vi "Range_Adjust.vi"(8 "error in (no error)":errorcluster, 11 ".NET Reference in":refnum<k24>) -> (0 "error out":errorcluster, 3 "Reference out":refnum<k24>)   [LabVIEW 2017]
doc: "OSU range adjust"
uses:
  D:/test/FULLband-sts/Fullband_Sample/DLL/InstrumentDLL.dll
  DLL/InstrumentDLL.dll
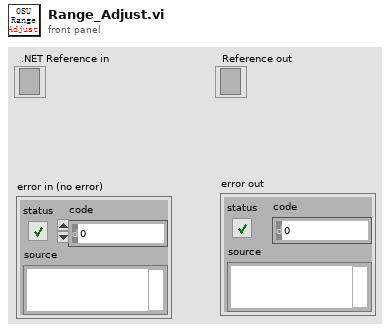
[diagram p1: front panel]
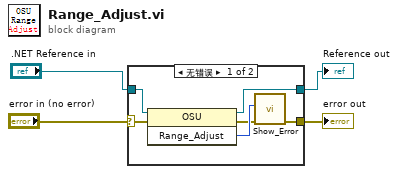
[diagram p0: block diagram]
diagram:
  n1 = case shown="无错误" "error in (no error)" {
    selector: "error in (no error)" -> [w8 w12]
    tunnel: ".NET Reference in" -> [w10 w11]
    tunnel: [w9 w11] -> w3
    tunnel: [w5 w12] -> w1
    frame No Error {
      n2 = invoke on="调用节点" class="OSU" method="Range_Adjust"(reference=w10, error in=w8) -> (reference out=w9:refnum<k24>, error out=w6:errorcluster, "Range_Adjust"=w7:i32)  [unwired: 1 in]
      n3 = call "Show_Error.vi"("error in (no error)"=w6, "Error"=w7) -> ("error out"=w5:errorcluster)  [unwired: 9 in]
    }
    frame Error {
    }
  }
  "error out" <- w1
  "Reference out" <- w3
